vi "ADC INL_sweep_triangle.vi"(8 "error in (no error)":errorcluster, 9 "Sequence parameters":string[][](array[string])=[["Min limit", "Max limit", "Register sheet file", "Register Sheet"], ["", "", "CC2600.xls", "TX_BLE;Trim"], ["Reg write (addr;value)", "Operating frequency [Hz]", "", ""], ["NA", "2.44G", "", ""]], 10 "Run type":i32, 11 "Method parameters":T3={"Dev"={"Do not disturb DUT"=FALSE, "XOSC"=32000000.0, "Board type"="", "EM"="", "Configure tempboard"=TRUE, "Device specific info"=[], "Generic Object"=refnum}, "Method"={"Run type"=1, "Test name"="Current LPM2 4", "Comment"="", "Results folder"="", "AFC"=enum."Off", "Method name"="Current LPM2 4", "Method results"={"Excel brief report"=FALSE, "Spotfire report"=FALSE, "Starfish report"=FALSE}, "Operator"="", "Reference time"=timestamp(0 s since 1904-01-01), "AFC delay"=0.0, "Initialization"=enum."Enabled", "MD5 Sum"="", "HW addon board"=enum."None", "AFC Regsheet"="", "AFC Regfile"=path "", "dummy"=0.0}, "Inst"={"Instr"={"PS1"={"Name"="", "GPIB address"="", "VISA session"=""}, "PS2"={"Name"="", "GPIB address"="", "VISA session"=""}, "TC1"={"Name"="", "GPIB address"="", "VISA session"=""}, "TC2"={"Name"="", "GPIB address"="", "VISA session"=""}, "SA1"={"Name"="", "GPIB address"="", "VISA session"=""}, "SA2"={"Name"="", "GPIB address"="", "VISA session"=""}, "SG1"={"Name"="", "GPIB address"="", "VISA session"=""}, "SG2"={"Name"="", "GPIB address"="", "VISA session"=""}, "SG3"={"Name"="", "GPIB address"="", "VISA session"=""}, "MI1"={"Name"="", "GPIB address"="", "VISA session"=""}, "MI2"={"Name"="", "GPIB address"="", "VISA session"=""}, "SW SA"={"Name"="", "Controller addr"=""}, "SW SG"={"Name"="", "Controller addr"=""}, "MI3"={"Name"="", "GPIB address"="", "VISA session"=""}}, "Switchbox"={"RF Path"=0, "Cal compensation"=enum."TX", "Switchbox gain mode"="", "State"=enum."TX"}, "Instr to control (i.e. SA1)"="Default", "Intrument info string"=""}, "Sequence parameters"=[["Weight", "Min Limit", "Max Limit", "Register Sheet", "", "", "", "", "", "", "", "", ""], ["Vital", "", "1", "LPM2", "", "", "", "", "", "", "", "", ""], ["Resolution", "Reg write (addr;value)", "Chip mode", "Range", "", "", "", "", "", "", "", "", ""], ["u", "NA", "", "auto", "", "", "", "", "", "", "", "", ""]], "Cond"={"Temp logged"=25.0, "VDD1_PS1_6V"=-999.0, "VDD2_PS1_25V"=-999.0, "VDD4_PS2_25V"=-999.0, "VDD3_PS2_6V"=-999.0}, "Meas config"={"X-axis inner loop index"=32000000, "Y-axis outer loop index"=32000000, "X-axis"=[], "Y-axis"=[], "X-axis array req size"=32000000, "Y-axis array req size"=32000000, "Param description"=[], "Use meas clust for reporting"=FALSE, "Parameter index (page)"=0, "X-axis name"="", "Y-axis name"=""}} {"Cond"."VDD3_PS2_6V" format="%.3f"; "Cond"."VDD4_PS2_25V" format="%.3f"; "Cond"."VDD2_PS1_25V" format="%.3f"; "Cond"."VDD1_PS1_6V" format="%.3f"; "Method"."dummy" format="%.1p"; "Method"."AFC delay" format="%.1p"; "Dev"."XOSC" format="%.3p"}) -> (0 "error out":errorcluster, 1 "End method error":T2, 2 "Short Results":string[](array[string])=["0.00", "0.00", "0.00", "0.00"], 3 "Result summary":string[][](array[string])=[["Critical", "Output Power@2405 MHz", "-3", "4", "dBm"], ["Critical", "Output Power@2410 MHz", "-3", "4", "dBm"]])   [LabVIEW 2019]
doc: "[AutoDocStart]Performs crystal accuracy measurements. Measures the offset from ideal frequency. Primarily used for tuning XOSC capacitors and verifying XOSC trims.\n\nSweeping parameters: operating frequency, OSC override value and VDDR level\n\nResults: Offset frequency in ppm[AutoDocEnd]"
uses:
  User Lib/Utilities/Cluster definitions/Method input.ctl
  User Lib/Utilities/Cluster definitions/Device specific info.ctl
  User Lib/Utilities/Controls/Automatic Frequency Compensation types.ctl
  User Lib/Utilities/Controls/Method Reports.ctl
  User Lib/Utilities/Cluster definitions/Method Initialization.ctl
  User Lib/Utilities/Controls/HW addon boards.ctl
  User Lib/Utilities/Cluster definitions/Instr clust.ctl
  User Lib/Utilities/Switchbox control/SwitchBox_State._ENUMctl.ctl
  User Lib/Utilities/Cluster definitions/End method error cluster.ctl
  User Lib/Utilities/Cluster definitions/DUT vdd control.ctl
  User Lib/Utilities/Cluster definitions/DUT VDD4.ctl
  User Lib/Utilities/Cluster definitions/DUT VDD3.ctl
  User Lib/Utilities/Cluster definitions/DUT VDD2.ctl
  User Lib/Utilities/Cluster definitions/DUT VDD1.ctl
  3a26386c-adf8-4bfd-9313-23d3b8777f38.vi
panel:
  in  "Tab Control":T1(tab)
  # "°C"
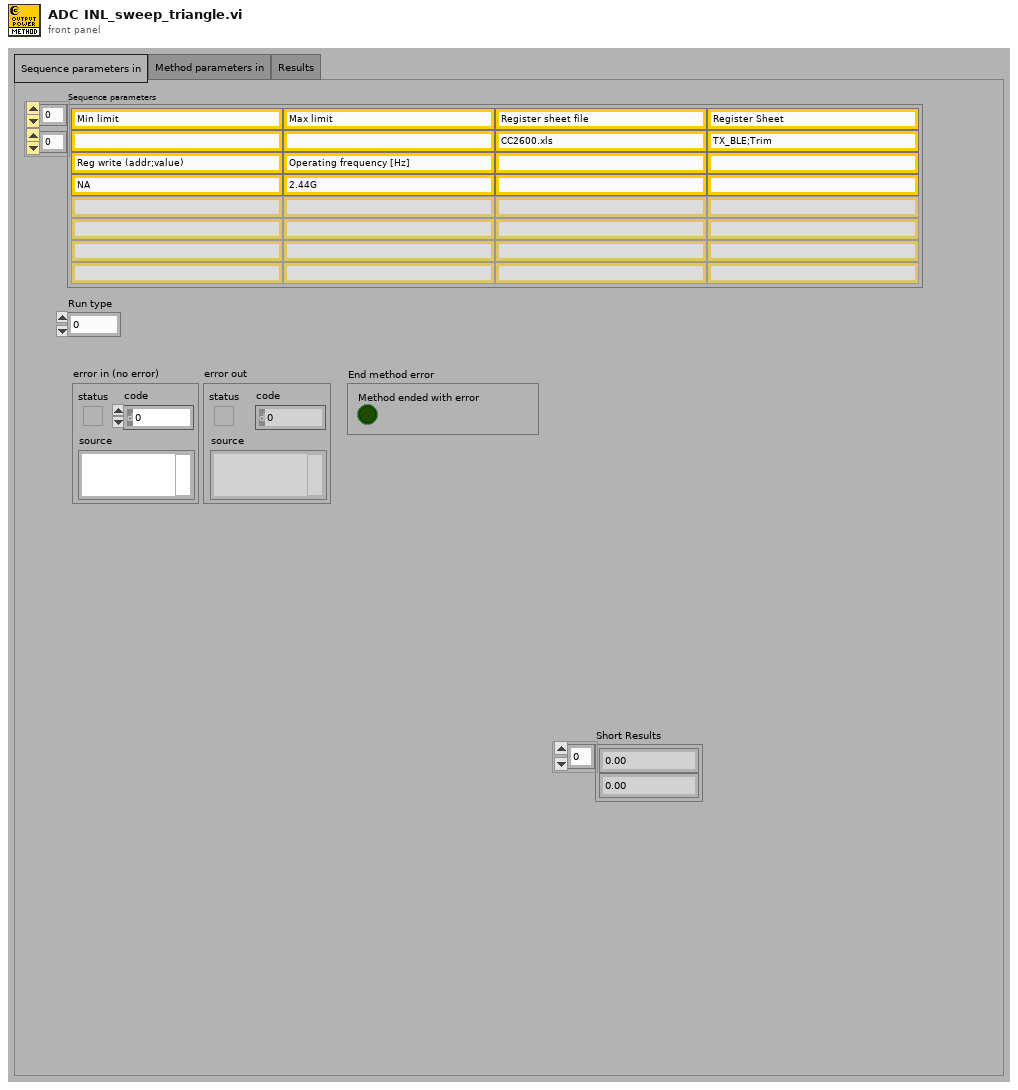
[diagram p1: front panel]
types:
  T1 = enum32{"Sequence parameters in", "Method parameters in", "Results"}
  T2 = typedef "End method error cluster.ctl" = cluster{"Method ended with error":bool}
  T3 = typedef "Method input.ctl" = cluster{"Dev":cluster{"Do not disturb DUT":bool, "XOSC":dbl, "Board type":string, "EM":string, "Configure tempboard":bool, "Device specific info":T4[], "Generic Object":refnum<class>}, "Method":cluster{"Run type":i32, "Test name":string, "Comment":string, "Results folder":string, "AFC":T5, "Method name":string, "Method results":T6, "Operator":string, "Reference time":timestamp, "AFC delay":dbl, "Initialization":T7, "MD5 Sum":string, "HW addon board":T8, "AFC Regsheet":string, "AFC Regfile":path, "dummy":dbl}, "Inst":T9, "Sequence parameters":string[][], "Cond":cluster{"Temp logged":dbl, "VDD1_PS1_6V":dbl, "VDD2_PS1_25V":dbl, "VDD4_PS2_25V":dbl, "VDD3_PS2_6V":dbl}, "Meas config":cluster{"X-axis inner loop index":i32, "Y-axis outer loop index":i32, "X-axis":string[], "Y-axis":string[], "X-axis array req size":i32, "Y-axis array req size":i32, "Param description":string[][], "Use meas clust for reporting":bool, "Parameter index (page)":i32, "X-axis name":string, "Y-axis name":string}}
  T4 = typedef "Device specific info.ctl" = cluster{"EM number":u8, "IP address":string, "Enabled":bool, "Slot no":u8, "RF path":u8, "EM name":string, "Wafer info":string, "AFC frequency ppm":dbl, "Register writes":string[][], "Meas data":string[][][], "Device comment":string}
  T5 = typedef "Automatic Frequency Compensation types.ctl" = enum16{"Off", "Compensate Instrument frequency", "Compensate DUT frequency", "Predictive - Compensate Instrument frequency", "Predictive - Compensate DUT frequency", "Do not skip re-init - Compensate Instrument frequency", "Do not skip re-init - Compensate DUT frequency"}
  T6 = typedef "Method Reports.ctl" = cluster{"Excel brief report":bool, "Spotfire report":bool, "Starfish report":bool}
  T7 = typedef "Method Initialization.ctl" = enum16{"Enabled", "Skip Instr and Device Init", "Enabled with Separate Flash", "Set PS, Device Init and Skip Instr Init", "Skip Device Init"}
  T8 = typedef "HW addon boards.ctl" = enum16{"None", "Current meas 5EM", "Stresstest 10EM"}
  T9 = typedef "Instr clust.ctl" = cluster{"Instr":cluster{"PS1":cluster{"Name":string, "GPIB address":string, "VISA session":refnum<visa-resource-name>}, "PS2":cluster{"Name":string, "GPIB address":string, "VISA session":refnum<visa-resource-name>}, "TC1":cluster{"Name":string, "GPIB address":string, "VISA session":refnum<visa-resource-name>}, "TC2":cluster{"Name":string, "GPIB address":string, "VISA session":refnum<visa-resource-name>}, "SA1":cluster{"Name":string, "GPIB address":string, "VISA session":refnum<visa-resource-name>}, "SA2":cluster{"Name":string, "GPIB address":string, "VISA session":refnum<visa-resource-name>}, "SG1":cluster{"Name":string, "GPIB address":string, "VISA session":refnum<visa-resource-name>}, "SG2":cluster{"Name":string, "GPIB address":string, "VISA session":refnum<visa-resource-name>}, "SG3":cluster{"Name":string, "GPIB address":string, "VISA session":refnum<visa-resource-name>}, "MI1":cluster{"Name":string, "GPIB address":string, "VISA session":refnum<visa-resource-name>}, "MI2":cluster{"Name":string, "GPIB address":string, "VISA session":refnum<visa-resource-name>}, "SW SA":cluster{"Name":string, "Controller addr":string}, "SW SG":cluster{"Name":string, "Controller addr":string}, "MI3":cluster{"Name":string, "GPIB address":string, "VISA session":refnum<visa-resource-name>}}, "Switchbox":cluster{"RF Path":i32, "Cal compensation":enum16{"TX", "RX", "Interferer", "No compensation", "Interferer2"}, "Switchbox gain mode":string, "State":T10}, "Instr to control (i.e. SA1)":string, "Intrument info string":string}
  T10 = typedef "SwitchBox_State._ENUMctl.ctl" = enum16{"TX", "RX", "SP:TX", "SP:RX", "SW:TX", "SW:RX"}
  T11 = typedef "DUT vdd control.ctl" = cluster{"VDD4 config":T12, "VDD3 config":T13, "VDD2 config":T14, "VDD1 config":T15}
  T12 = typedef "DUT VDD4.ctl" = u16
  T13 = typedef "DUT VDD3.ctl" = u16
  T14 = typedef "DUT VDD2.ctl" = u16
  T15 = typedef "DUT VDD1.ctl" = u16
  T16 = enum32{"NI Card Settings", "Memory Read Setting", "DC Capture", "ADC Ramp", "ADC Sine", "SNR", "Cap Calibration"}
  T17 = enum32{"Read from Memory", "Read .dat file", "NI Card Capture", "None"}
  T18 = cluster{"Path to Save plot":path, "Path to Raw Data plot":path}
  T19 = cluster{"Save INL/DNL Plot(Ramp)":bool, "Save SNR Plot":bool, "Save INL/DNL Plot(Sine)":bool, "Save INL/DNL Raw Data(Ramp)":bool, "Save SNR Raw Data":bool, "Save INL/DNL Raw Data(Sine)":bool, "Save DC Raw data":bool, "Save  Raw Data(Sine)":bool}
  T20 = cluster{"Min INL":dbl, "Max INL":dbl, "Min DNL":dbl, "Max DNL":dbl, "INL Range":dbl, "DNL Range":dbl, "Avg Hits/Code":dbl}
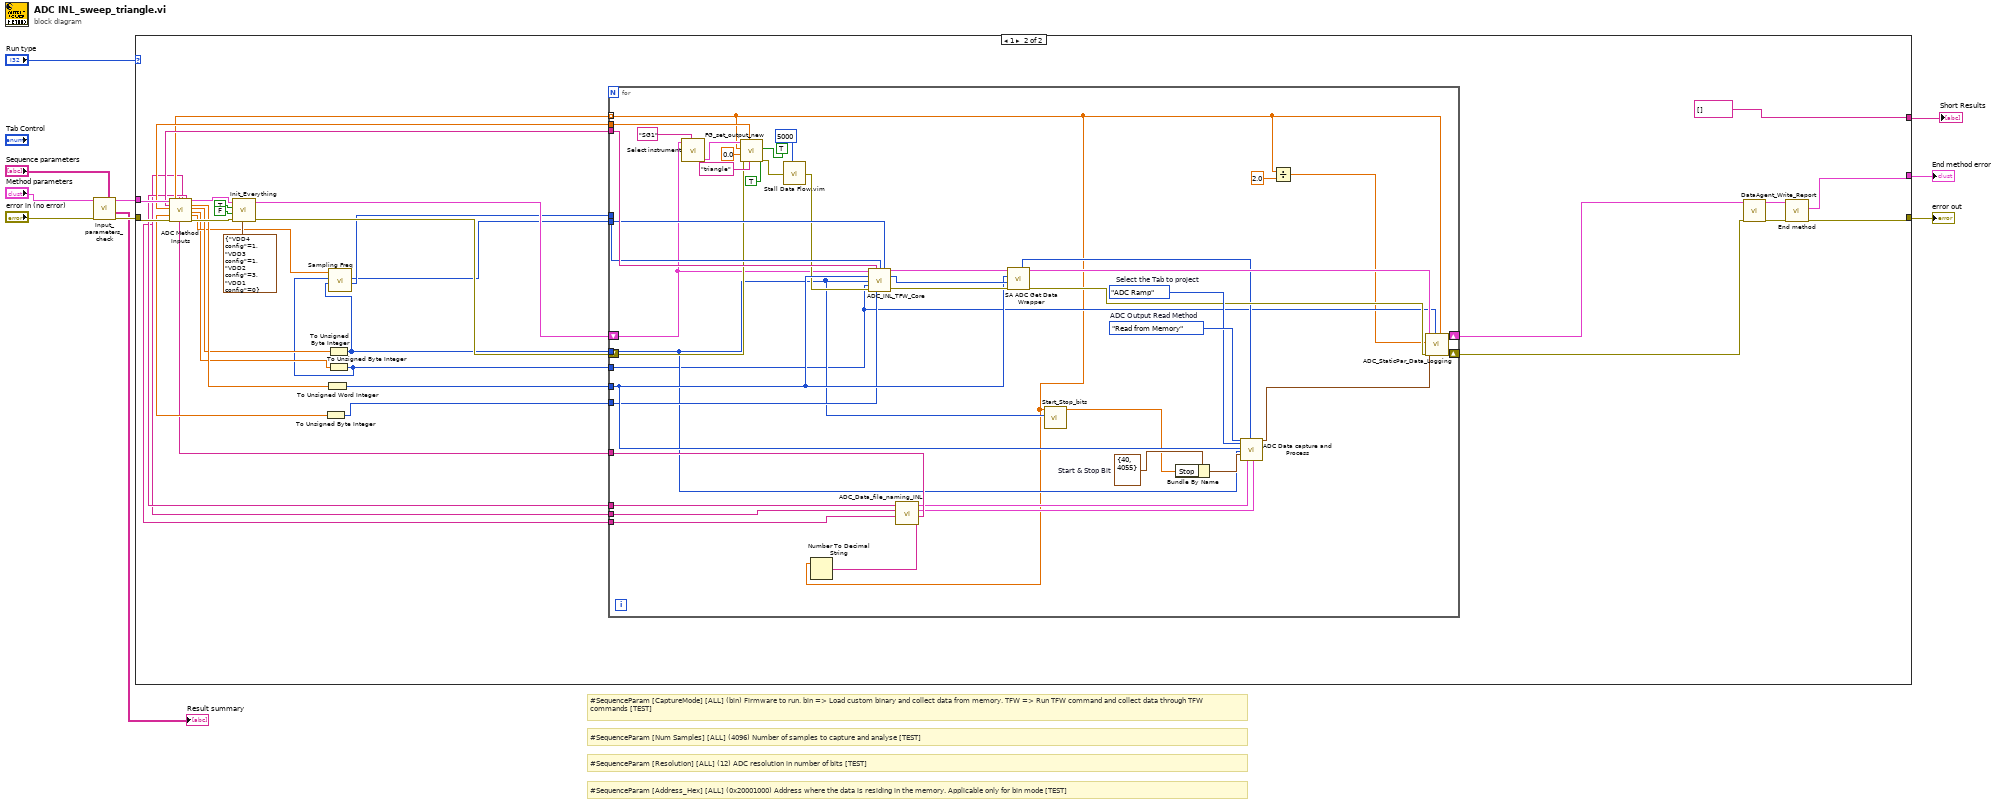
[diagram p0: block diagram]
diagram:
  # "#SequenceParam [Num Samples] [ALL] (4096) Number of samples to capture and analyse [TEST]"
  # "#SequenceParam [CaptureMode] [ALL] (bin) Firmware to run. bin => Load custom binary and collect data from memory. TFW => Run TFW command and collect data through TFW commands [TEST]"
  # "#SequenceParam [Address_Hex] [ALL] (0x20001000) Address where the data is residing in the memory. Applicable only for bin mode [TEST]"
  # "#SequenceParam [Resolution] [ALL] (12) ADC resolution in number of bits [TEST]"
  n1 = call "Input_parameters_check.vi"("Sequence parameters"="Sequence parameters", "error in"="error in (no error)", "Method cluster in"="Method parameters") -> ("error out"=w9:errorcluster, "Result summary"=→"Result summary":string[][], "Method cluster out"=w5:T3)  [unwired: 6 in]
  n2 = case shown="1" "Run type" {
    tunnel: w9 -> [w11 w34]
    tunnel: [w11 w45] -> w10
    tunnel: w5 -> [_ w35]
    tunnel: [_ w44] -> w4
    tunnel: [_ string[] []] -> w1
    frame 0, Default {
      # "Run type 0 is only for formatting the result summary"
    }
    frame 1 {
      n3 = call "ADC Method Inputs.vi"("Method cluster in"=w35, "error in (no error)"=w34) -> ("Capture Mode"=w21:string, "Signal Freq"=w17:dbl, "ADC Chnl No."=w27:dbl, "Input Voltage"=w16:dbl[], "Sampling Freq String"=w13:string, "Chnl No. string"=w12:string, "Resolution String"=w14:string, "Voltage Ref String"=w15:string, "Method cluster out"=w32:T3, "Num Samples"=w31:dbl, "Resolution"=w30:dbl, "Voltage Ref"=w28:dbl, "Sampling Freq"=w29:dbl, "error out"=w33:errorcluster)  [unwired: 3 in, 1 out]
      n4 = call "Init_Everything.vi"("VDD config"=T11 {"VDD4 config"=1, "VDD3 config"=1, "VDD2 config"=3, "VDD1 config"=0}, "error in"=w33, "Support current measurement?"=FALSE, "Override VDD Config"=TRUE, "Method cluster In"=w32) -> ("error out"=w25:errorcluster, "Method cluster out"=w26:T3)  [unwired: 3 in, 2 out]
      n5 = To Unsigned Byte Integer(number=w27) -> (unsigned 8bit integer=w22:u8)
      n6 = To Unsigned Word Integer(number=w31) -> (unsigned 16bit integer=w24:u16)
      n7 = To Unsigned Byte Integer(number=w30) -> (unsigned 8bit integer=w23:u8)
      n8 = To Unsigned Byte Integer(number=w28) -> (unsigned 8bit integer=w18:u8)
      n9 = call "Sampling Freq.vi"("Resolution"=w23, "Voltage Ref"=w18, "Sampling Freq"=w29) -> ("LGPT Count"=w20:u16, "SCOMP"=w19:u16)  [unwired: 7 in]
      n10 = for {
        tunnel: w24 -> [w78]
        tunnel: w23 -> [w51]
        tunnel: w18 -> [w49]
        tunnel: w22 -> [w77]
        tunnel: w21 -> [w76]
        tunnel: w20 -> [w75]
        tunnel: w19 -> [w74]
        shift-right: [w83] -> w39
        shift-left: w26 -> [w68]
        shift-right: [w82] -> w38
        shift-left: w25 -> [w71]
        tunnel: w16 -> [w48] mode=indexing
        tunnel: w17 -> [w65]
        tunnel: w15 -> [w60]
        tunnel: w14 -> [w62]
        tunnel: w13 -> [w61]
        tunnel: w12 -> [w59]
        w55 = cluster{"Start":i32, "Stop":i32} {"Start"=40, "Stop"=4055}  # Start & Stop Bit
        w87 = T16."ADC Ramp"  # Select the Tab to project
        w88 = T17."Read from Memory"  # ADC Output Read Method
        n11 = call "Select instrument.vi"("Instr.Instr to control (i.e. SA1)"="SG1", "Method cluster in"=w68) -> ("Instr out"=w73:T9)  [unwired: 7 in, 2 out]
        n12 = call "FG_set_output_new.vi"("High impedance (T)"=TRUE, "Enable Output?"=TRUE, "Function (DC, Sine, Square, Triangle, Ramp up, Ramp down, Pulse)"="triangle", "Frequency [Hz]"=w65, "error in"=w71, "Low voltage"=0.0, "High voltage (or DC)"=w48, "InstrCluster in"=w73) -> ("error out"=w70:errorcluster)  [unwired: 2 in, 1 out]
        n13 = call "Stall Data Flow.vim"("value in"=w70, "milliseconds to wait"=u32 5000) -> ("value out"=w69:errorcluster)  [unwired: 1 out]
        n14 = Number To Decimal String(number=w48) -> (decimal integer string=w50:string)  [unwired: 1 in]
        n15 = call "ADC_INL_TFW_Core.vi"("Method cluster in"=w68, "Capture Mode"=w76, "LGPT Count"=w75, "SCOMP"=w74, "No. Samples"=w78, "Resolution"=w51, "Voltage Ref"=w49, "error in"=w69, "ADC Chnl No."=w77) -> ("Method cluster out"=w53:T3, "ResPar[0] Data Address"=w79:u32, "error out"=w80:errorcluster)  [unwired: 3 in, 1 out]
        n16 = call "ADC_Data_file_naming_INL.vi"("Amplitude (Vpp)"=w50, "ADC Chn. No"=w59, "Sampling Freq String"=w61, "Resolution String"=w62, "Voltage Ref String"=w60) -> ("path to save"=w57:T18, "Save data"=w58:T19)  [unwired: 5 in]
        n17 = call "SA ADC Get Data Wrapper.vi"("error in"=w80, "Data Address"=w79, "Num Samples"=w78, "Method cluster in"=w53) -> ("error out"=w86:errorcluster, "output cluster"=w85:T3, "ADC samples"=w84:u32[])  [unwired: 2 in, 3 out]
        n18 = call "Start_Stop_bits.vi"("Resolution"=w51, "Input Amplitude"=w48) -> ("Stop Bit"=w52:dbl)  [unwired: 9 in]
        n19 = Bundle By Name(cluster=w55, "Stop"=w52) -> (w54:cluster{"Start":i32, "Stop":i32})
        n20 = call "ADC Data capture and Process.vi"("ADC Output Read Method"=w88, "Select the Tab to project"=w87, "No.of samples"=w78, "Resolution"=w51, "Start & Stop Bit"=w54, "Save data"=w58, "Input Waveform"=w84, "path to save"=w57) -> ("Static Parameters (Ramp)"=w81:T20)  [unwired: 14 in, 5 out]
        n21 = Divide(x=w48, y=2.0) -> (x/y=w46:dbl)
        n22 = call "ADC_StaticPar_Data_Logging.vi"("Offset (V)"=w46, "Amplitude (Vpp)"=w48, "Ref Voltage"=w49, "error in (no error)"=w86, "Static Parameters (Ramp)"=w81, "output cluster"=w85) -> ("error out"=w82:errorcluster, "Method cluster out"=w83:T3)  [unwired: 4 in]
      }
      n23 = call "DataAgent_Write_Report.vi"("error in (no error)"=w38, "Method cluster in"=w39) -> ("error out"=w42:errorcluster, "Method cluster out"=w41:T3)  [unwired: 8 in]
      n24 = call "End method.vi"("error in"=w42, "Method cluster in"=w41) -> ("error out"=w45:errorcluster, "End method error"=w44:T2)  [unwired: 7 in, 1 out]
    }
  }
  "error out" <- w10
  "End method error" <- w4
  "Short Results" <- w1
